vi "StressTankDrive.vi"(8 "error in (no error)":errorcluster, 10 "Num instructions":i32, 11 "TankDriveQueue":refnum<queue>) -> (0 "error out":errorcluster)   [LabVIEW 2013]
doc: "Stress test for fire pneumatic."
uses:
  QueueInstruction.ctl
  SubsystemEnum.ctl
  ActionEnum.ctl
  TankDriveInstruction.ctl
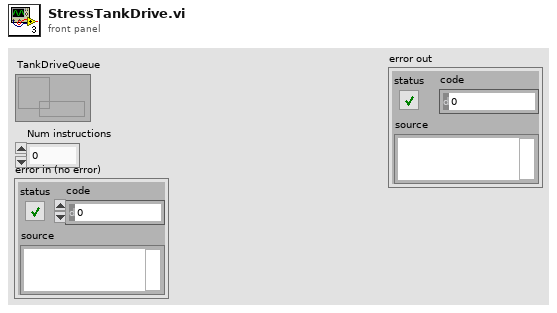
[diagram p1: front panel]
types:
  T1 = typedef "TankDriveInstruction.ctl" = cluster{"LeftMotorValue":dbl, "RightMotorValue":dbl, "HalfSpeed":bool}
  T2 = typedef "QueueInstruction.ctl" = cluster{"Data":variant, "Subsystem":T3, "Action":T4}
  T3 = typedef "SubsystemEnum.ctl" = enum16{"TankDrive", "FirePneumatic", "Climber", "ClimbWeight", "ShooterAngle"}
  T4 = typedef "ActionEnum.ctl" = enum16{"Init", "SetValue"}
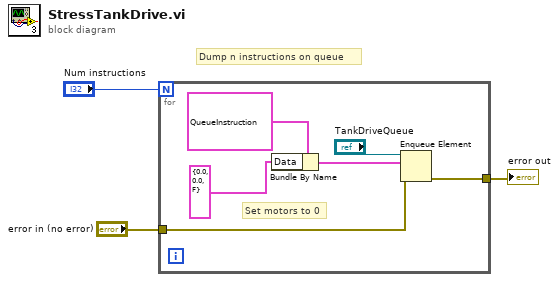
[diagram p0: block diagram]
diagram:
  # "Dump n instructions on queue"
  n1 = for {
    N: "Num instructions" -> [_]
    tunnel: "error in (no error)" -> [w6]
    tunnel: [w5] -> w1
    # "Set motors to 0"
    n2 = Bundle By Name(cluster=T2 {"Data"=variant, "Subsystem"=enum."TankDrive", "Action"=enum."SetValue"}, "Data"=T1 {"LeftMotorValue"=0.0, "RightMotorValue"=0.0, "HalfSpeed"=FALSE} ("TankDriveInstruction")) -> (w7:T2)
    n3 = Enqueue Element(queue="TankDriveQueue", element=w7, error in (no error)=w6) -> (error out=w5:errorcluster)  [unwired: 1 in, 2 out]
  }
  "error out" <- w1
